vi "HFRR ADV v019 new software.vi"() -> ()   [LabVIEW 2025] (continued)
        n906 = call <vilib>:"Clear Errors.vi"("error in (no error)"=w1070) -> ("error out"=w1069:errorcluster)  [unwired: 5 in, 1 out]
        n907 = call "IMAGE ANALYSIS.vi"("Enum"=POST_ANALYSIS_ENUM."SHOW UI", "error in"=w1069) -> ("error out"=w1067:errorcluster)  [unwired: 8 in, 1 out]
        n908 = local write "Zoom Factore"(100.0 ("Zoom Factore")) -> ()
      }
    }
    n909 = case shown="True" w758 {
      selector: w758 -> [_ w1046]
      tunnel: w750 -> [w1043 w1051]
      tunnel: [w1043 w1045] -> _
      frame False {
      }
      frame True {
        n910 = Not(x=w1046) -> (.not. x?=w1044:bool)
        n911 = local read "Zoom Factore"() -> (w1049:dbl)
        n912 = local write "OUT"(w1044) -> ()
        n913 = call "IMAGE ANALYSIS.vi"("Enum"=POST_ANALYSIS_ENUM."ZOOM OUT", "error in"=w1051) -> ("error out"=w1045:errorcluster)  [unwired: 8 in, 1 out]
        n914 = Divide(x=w1049, y=1.2) -> (x/y=w1047:dbl)
        n915 = local write "Zoom Factore"(w1047) -> ()
      }
    }
    n916 = case shown="True" w759 {
      selector: w759 -> [_ w1055]
      tunnel: w750 -> [w1052 w1060]
      tunnel: [w1052 w1053] -> _
      frame False {
      }
      frame True {
        n917 = Not(x=w1055) -> (.not. x?=w1054:bool)
        n918 = local read "Zoom Factore"() -> (w1058:dbl)
        n919 = local write "In"(w1054) -> ()
        n920 = call "IMAGE ANALYSIS.vi"("Enum"=POST_ANALYSIS_ENUM."ZOOM IN", "error in"=w1060) -> ("error out"=w1053:errorcluster)  [unwired: 8 in, 1 out]
        n921 = Multiply(x=w1058, y=1.2) -> (x*y=w1056:dbl)
        n922 = local write "Zoom Factore"(w1056) -> ()
      }
    }
    n923 = case shown="True" w755 {
      selector: w755 -> [_ w1027]
      tunnel: w750 -> [w1025 w1029]
      tunnel: [w1025 w1028] -> _
      frame False {
      }
      frame True {
        n924 = Not(x=w1027) -> (.not. x?=w1026:bool)
        n925 = local write "Clear ROI Tool"(w1026) -> ()
        n926 = call "IMAGE ANALYSIS.vi"("Enum"=POST_ANALYSIS_ENUM."CLEAR ROI", "error in"=w1029) -> ("error out"=w1028:errorcluster)  [unwired: 8 in, 1 out]
      }
    }
    n927 = case shown="True" w757 {
      selector: w757 -> [_ w1039]
      tunnel: w750 -> [w1037 w1042]
      tunnel: [w1037 w1040] -> _
      frame False {
      }
      frame True {
        n928 = Not(x=w1039) -> (.not. x?=w1038:bool)
        n929 = local write "line tool"(w1038) -> ()
        n930 = call "IMAGE ANALYSIS.vi"("Enum"=POST_ANALYSIS_ENUM."DRAW LINE", "error in"=w1042) -> ("error out"=w1040:errorcluster)  [unwired: 8 in, 1 out]
      }
    }
    n931 = case shown="True" w756 {
      selector: w756 -> [_ w1033]
      tunnel: w750 -> [w1031 w1035]
      tunnel: [w1031 w1034] -> _
      frame False {
      }
      frame True {
        n932 = Not(x=w1033) -> (.not. x?=w1032:bool)
        n933 = local write "Rectangle Tool"(w1032) -> ()
        n934 = call "IMAGE ANALYSIS.vi"("Enum"=POST_ANALYSIS_ENUM."DRAW REC", "error in"=w1035) -> ("error out"=w1034:errorcluster)  [unwired: 8 in, 1 out]
      }
    }
    n935 = local read "SCAR MEASURMENT"() -> (w743:enum32{"Auto Scar", "Manual Scar"})
    n936 = local read "Fit to Screen Tool"() -> (w752:bool)
    n937 = local read "Resize Tool"() -> (w751:bool)
    n938 = case shown="\"Manual Scar\", Default" w743 {
      frame "Auto Scar" {
        n939 = property on="Cap Live Image" class="Bool (strict)"("BoolText.Text"="Report" ("Boolean Text.Text")) -> ()  [unwired: 2 in, 2 out]
      }
      frame "Manual Scar", Default {
        n940 = property on="Cap Live Image" class="Bool (strict)"("BoolText.Text"="Save Image" ("Boolean Text.Text")) -> ()  [unwired: 2 in, 2 out]
      }
    }
    n941 = local read "ROI Color Tool"() -> (w753:bool)
    n942 = local read "Pan Tool"() -> (w754:bool)
    n943 = case shown="True" w754 {
      selector: w754 -> [_ w1021]
      tunnel: w750 -> [w1019 w1023]
      tunnel: [w1019 w1022] -> _
      frame False {
      }
      frame True {
        n944 = Not(x=w1021) -> (.not. x?=w1020:bool)
        n945 = call "IMAGE ANALYSIS.vi"("Enum"=POST_ANALYSIS_ENUM."PAN", "error in"=w1023) -> ("error out"=w1022:errorcluster)  [unwired: 8 in, 1 out]
        n946 = local write "Pan Tool"(w1020) -> ()
      }
    }
    n947 = case shown="True" w751 {
      selector: w751 -> [_ w1005]
      tunnel: w750 -> [w1000 w1002]
      tunnel: [w1000 w1001] -> _
      frame False {
      }
      frame True {
        n948 = Not(x=w1005) -> (.not. x?=w1004:bool)
        n949 = local write "Resize Tool"(w1004) -> ()
        n950 = call "IMAGE ANALYSIS.vi"("Enum"=POST_ANALYSIS_ENUM."RESIZE MODE", "error in"=w1002) -> ("error out"=w1001:errorcluster)  [unwired: 8 in, 1 out]
      }
    }
    n951 = case shown="True" w752 {
      selector: w752 -> [_ w1010]
      tunnel: [w1006 w1011] -> _
      tunnel: w750 -> [w1006 w1009]
      frame False {
      }
      frame True {
        n952 = Not(x=w1010) -> (.not. x?=w1008:bool)
        n953 = local write "Zoom Factore"(100.0 ("Zoom Factore")) -> ()
        n954 = local write "Fit to Screen Tool"(w1008) -> ()
        n955 = call "IMAGE ANALYSIS.vi"("Enum"=POST_ANALYSIS_ENUM."FIT", "error in"=w1009) -> ("error out"=w1011:errorcluster)  [unwired: 8 in, 1 out]
      }
    }
    n956 = case shown="True" w753 {
      selector: w753 -> [_ w1016]
      tunnel: [w1013 w1017] -> _
      tunnel: w750 -> [w1013 w1014]
      frame False {
      }
      frame True {
        n957 = Not(x=w1016) -> (.not. x?=w1015:bool)
        n958 = local write "ROI Color Tool"(w1015) -> ()
        n959 = call "IMAGE ANALYSIS.vi"("Enum"=POST_ANALYSIS_ENUM."SET ROI COLOR", "error in"=w1014) -> ("error out"=w1017:errorcluster)  [unwired: 8 in, 1 out]
      }
    }
    n960 = local read "Quit"() -> (w767:bool)
  }
  n961 = while {
    stop <- w1101 stop-if-true
    n962 = local read "Image Path"() -> (w1104:path)
    n963 = local read "Print 3"() -> (w1107:bool)
    n964 = Equal?(x=w1104, y=path "") -> (x = y?=w1103:bool)
    n965 = Not(x=w1103) -> (.not. x?=w1102:bool)
    n966 = property on="Print 3" class="Bool (strict)"("Visible"=w1102) -> ()  [unwired: 2 in, 2 out]
    n967 = case shown="True" w1107 {
      frame False {
        n968 = local write "Rd"(TRUE ("Boolean 7")) -> ()
      }
      frame True {
        n969 = flat-sequence {
          tunnel: [w1147] -> w1115
          tunnel: [w1134] -> w1113
          tunnel: [w1144] -> w1109
          tunnel: w1115 -> [w1156]
          tunnel: [w1156] -> w1114
          tunnel: w1113 -> [w1155]
          tunnel: [w1155] -> w1112
          tunnel: [w1153] -> w1111
          tunnel: [w1152] -> w1110
          tunnel: w1109 -> [w1152]
          tunnel: w1114 -> [w1158]
          tunnel: w1112 -> [w1159]
          tunnel: w1111 -> [_]
          tunnel: w1110 -> [w1157]
          frame #0 {
            n970 = case shown="True" "Rd" {
              frame False {
              }
              frame True {
                n971 = while {
                  tunnel: "abcdefABCDEF" ("string 2") -> [w1126]
                  shift-right: [w1124] -> w1118
                  shift-left: "" -> [w1123]
                  i -> [w1133]
                  stop <- w1132 stop-if-true
                  n972 = Random Number (0-1)() -> (number: 0 to 1=w1127:dbl)
                  n973 = Multiply(x=w1127, y=62.0) -> (x*y=w1129:dbl)
                  n974 = Decrement(x="Length 2") -> (x-1=w1122:i16)
                  n975 = To Word Integer(number=w1129) -> (16bit integer=w1130:i16)
                  n976 = String Subset(string=w1126, offset (0)=w1130, length (rest)=1 ("length (rest)")) -> (substring=w1125:string)
                  n977 = Greater Or Equal?(x=w1133, y=w1122) -> (x >= y?=w1132:bool)
                  n978 = Concatenate Strings(w1125, w1123) -> (w1124:string)
                }
                "String 10" <- w1118
                n979 = local write "Rd"(FALSE ("Boolean 7")) -> ()
              }
            }
          }
          frame #1 {
            w1145 = "_resized.jpg" ("command line")
            (unwired) ".jpg -resize 320x240 " ("string")
            (unwired) "Choose an Image File" ("prompt")
            # "-resize 1798x425"
            n980 = local read "Image Path"() -> (w1139:path)
            n981 = Strip Path(path=w1139) -> (stripped path=w1134:path, name=w1135:string)
            n982 = Match Pattern(string=w1135, regular expression=".jpg") -> (before substring=→"before substring 2":string, after substring=→"after substring":string)  [unwired: 1 in, 2 out]
            n983 = Match Pattern(string=w1135, regular expression="\\") -> (before substring=w1141:string)  [unwired: 1 in, 3 out]
            n984 = Match Pattern(string=w1141, regular expression=".jpg") -> (before substring=w1140:string)  [unwired: 1 in, 3 out]
            n985 = Concatenate Strings("cmd /c convert " ("string"), w1140, ".jpg -resize 320x240  " ("command line"), w1140, w1145) -> (w1148:string)
            n986 = call <vilib>:"System Exec.vi"("run minimized? (F)"=TRUE, "wait until completion? (T)"=TRUE, "working directory"=w1134, "command line"=w1148) -> ("error out"=w1147:errorcluster)  [unwired: 4 in, 3 out]
            "error out 2" <- w1147
            n987 = Concatenate Strings(w1140, w1145) -> (w1144:string)
          }
          frame #2 {
            n988 = Wait (ms)(milliseconds to wait=u32 2000 ("millisecond timer value")) -> (millisecond timer value=w1153:u32)
          }
          frame #3 {
            n989 = case shown="No Error" w1158 {
              tunnel: w1159 -> [w1162 _]
              tunnel: w1157 -> [w1160 _]
              frame No Error {
                (unwired) ".jpg" ("string")
                n990 = Path To String(path=w1162) -> (string=w1166:string)
                n991 = Concatenate Strings(w1166, "\\" ("string"), w1160) -> (w1165:string)
                n992 = String To Path(string=w1165) -> (path=w1164:path)
                n993 = call <vilib>:"Read JPEG File.vi"("path to JPEG file"=w1164) -> ("image data"=w1168:T16)  [unwired: 8 in, 2 out]
                "image data" <- w1168
                n994 = local write "Print 3"(FALSE ("Print 2")) -> ()
                n995 = call <vilib>:"Draw Flattened Pixmap.vi"("image data"=w1168) -> ("new picture"=→"new picture":picture)  [unwired: 8 in]
              }
              frame Error {
              }
            }
          }
        }
      }
    }
    n996 = Wait (ms)(milliseconds to wait=u32 20 ("millisecond timer value")) -> ()  [unwired: 1 out]
    n997 = local read "Quit"() -> (w1101:bool)
  }
  n998 = while {
    tunnel: w35 -> [_]
    tunnel: w19 -> [_]
    stop <- w1199 stop-if-true
    # "New Adv Logics"
    n999 = local read "Main Tab"() -> (w1179:T2)
    n1000 = local read "Main Tab"() -> (w1197:T2)
    n1001 = local read "Sign In"() -> (w1196:bool)
    n1002 = case shown="\"Adv Scar\"" w1179 {
      frame "HOME", Default {
        n1003 = local read "LIVE FEED MIN TEMP"() -> (w1332:bool)
        n1004 = local write "LIVE FEED MAX TEMP"(TRUE ("LIVE FEED MAX TEMP")) -> ()
        n1005 = local read "CAMERA ROI MIN TEMP"() -> (w1330:bool)
        n1006 = case shown="True" w1332 {
          selector: w1332 -> [_ w1339]
          frame False {
          }
          frame True {
            n1007 = Not(x=w1339) -> (.not. x?=w1338:bool)
            n1008 = local write "LIVE FEED MIN TEMP"(w1338) -> ()
            n1009 = call "CAMERA LIVE FEED FGV.vi"("Enum - Menu"=CAMERA_LIVE_FEED_ENUM."CAMERA MINIMIZE") -> ()  [unwired: 9 in, 2 out]
          }
        }
        n1010 = case shown="True" w1330 {
          selector: w1330 -> [_ w1336]
          frame False {
          }
          frame True {
            n1011 = Not(x=w1336) -> (.not. x?=w1335:bool)
            n1012 = local write "CAMERA ROI MIN TEMP"(w1335) -> ()
            n1013 = call "IMAGE ANALYSIS.vi"("Enum"=POST_ANALYSIS_ENUM."MINIMIZE UI") -> ()  [unwired: 9 in, 2 out]
          }
        }
        n1014 = local write "CAMERA ROI MAX TEMP"(TRUE ("CAMERA ROI MAX TEMP")) -> ()
      }
      frame "Test Setup" {
        n1015 = local read "LIVE FEED MIN TEMP"() -> (w1342:bool)
        n1016 = local read "CAMERA ROI MIN TEMP"() -> (w1340:bool)
        n1017 = local write "LIVE FEED MAX TEMP"(TRUE ("LIVE FEED MAX TEMP")) -> ()
        n1018 = case shown="True" w1342 {
          selector: w1342 -> [_ w1349]
          frame False {
          }
          frame True {
            n1019 = Not(x=w1349) -> (.not. x?=w1348:bool)
            n1020 = local write "LIVE FEED MIN TEMP"(w1348) -> ()
            n1021 = call "CAMERA LIVE FEED FGV.vi"("Enum - Menu"=CAMERA_LIVE_FEED_ENUM."CAMERA MINIMIZE") -> ()  [unwired: 9 in, 2 out]
          }
        }
        n1022 = case shown="True" w1340 {
          selector: w1340 -> [_ w1346]
          frame False {
          }
          frame True {
            n1023 = Not(x=w1346) -> (.not. x?=w1345:bool)
            n1024 = local write "CAMERA ROI MIN TEMP"(w1345) -> ()
            n1025 = call "IMAGE ANALYSIS.vi"("Enum"=POST_ANALYSIS_ENUM."MINIMIZE UI") -> ()  [unwired: 9 in, 2 out]
          }
        }
        n1026 = local write "CAMERA ROI MAX TEMP"(TRUE ("CAMERA ROI MAX TEMP")) -> ()
      }
      frame "Acquire" {
        n1027 = local read "LIVE FEED MIN TEMP"() -> (w1352:bool)
        n1028 = local write "LIVE FEED MAX TEMP"(TRUE ("LIVE FEED MAX TEMP")) -> ()
        n1029 = local read "CAMERA ROI MIN TEMP"() -> (w1350:bool)
        n1030 = case shown="True" w1352 {
          selector: w1352 -> [_ w1359]
          frame False {
          }
          frame True {
            n1031 = Not(x=w1359) -> (.not. x?=w1358:bool)
            n1032 = local write "LIVE FEED MIN TEMP"(w1358) -> ()
            n1033 = call "CAMERA LIVE FEED FGV.vi"("Enum - Menu"=CAMERA_LIVE_FEED_ENUM."CAMERA MINIMIZE") -> ()  [unwired: 9 in, 2 out]
          }
        }
        n1034 = case shown="True" w1350 {
          selector: w1350 -> [_ w1356]
          frame False {
          }
          frame True {
            n1035 = Not(x=w1356) -> (.not. x?=w1355:bool)
            n1036 = local write "CAMERA ROI MIN TEMP"(w1355) -> ()
            n1037 = call "IMAGE ANALYSIS.vi"("Enum"=POST_ANALYSIS_ENUM."MINIMIZE UI") -> ()  [unwired: 9 in, 2 out]
          }
        }
        n1038 = local write "CAMERA ROI MAX TEMP"(TRUE ("CAMERA ROI MAX TEMP")) -> ()
      }
      frame "Adv Scar" {
        n1039 = local read "CAMERA ROI MIN TEMP"() -> (w1360:bool)
        n1040 = case shown="True" "LIVE FEED MAX TEMP" {
          selector: "LIVE FEED MAX TEMP" -> [_ w1381]
          frame False {
          }
          frame True {
            n1041 = Not(x=w1381) -> (.not. x?=w1380:bool)
            n1042 = local write "LIVE FEED MAX TEMP"(w1380) -> ()
            n1043 = call "CAMERA LIVE FEED FGV.vi"("Enum - Menu"=CAMERA_LIVE_FEED_ENUM."CAMERA RESTORE") -> ("error out"=w1371:errorcluster)  [unwired: 9 in, 1 out]
            n1044 = Type Cast(type=30, x=0) -> (*(type *) &x=w1375:i32)
            n1045 = Add(x=w1375, y=48) -> (x+y=w1376:i32)
            n1046 = call "CAMERA LIVE FEED FGV.vi"("Enum - Menu"=CAMERA_LIVE_FEED_ENUM."CAMERA MODE SET", "error in (no error)"=w1371, "CAMERA MODE"=w1376) -> ("error out"=w1368:errorcluster)  [unwired: 7 in, 1 out]
            n1047 = call "CAMERA LIVE FEED FGV.vi"("Enum - Menu"=CAMERA_LIVE_FEED_ENUM."CAMERA GRAY", "error in (no error)"=w1368) -> ("error out"=w1367:errorcluster)  [unwired: 8 in, 1 out]
            n1048 = call "LIST FILE NAMES.vi"("error in (no error)"=w1367) -> ("error out"=w1377:errorcluster, "filenames"=w1378:string[])  [unwired: 9 in]
            n1049 = property on="FILE 3" class="CmbBox"(error in=w1377, "Strings[]"=w1378) -> ()  [unwired: 1 in, 2 out]
          }
        }
        n1050 = case shown="True" w1360 {
          selector: w1360 -> [_ w1366]
          frame False {
          }
          frame True {
            n1051 = Not(x=w1366) -> (.not. x?=w1365:bool)
            n1052 = local write "CAMERA ROI MIN TEMP"(w1365) -> ()
            n1053 = call "IMAGE ANALYSIS.vi"("Enum"=POST_ANALYSIS_ENUM."MINIMIZE UI") -> ()  [unwired: 9 in, 2 out]
          }
        }
        n1054 = local write "CAMERA ROI MAX TEMP"(TRUE ("CAMERA ROI MAX TEMP")) -> ()
        "LIVE FEED MIN TEMP" <- TRUE ("LIVE FEED MIN TEMP")
      }
      frame "Adv Scar Report" {
        n1055 = local read "CAMERA ROI MAX TEMP"() -> (w1382:bool)
        n1056 = local read "LIVE FEED MIN TEMP"() -> (w1384:bool)
        n1057 = local write "LIVE FEED MAX TEMP"(TRUE ("LIVE FEED MAX TEMP")) -> ()
        n1058 = case shown="True" w1384 {
          selector: w1384 -> [_ w1393]
          frame False {
          }
          frame True {
            n1059 = Not(x=w1393) -> (.not. x?=w1392:bool)
            n1060 = local write "LIVE FEED MIN TEMP"(w1392) -> ()
            n1061 = call "CAMERA LIVE FEED FGV.vi"("Enum - Menu"=CAMERA_LIVE_FEED_ENUM."CAMERA MINIMIZE") -> ()  [unwired: 9 in, 2 out]
          }
        }
        n1062 = case shown="True" w1382 {
          selector: w1382 -> [_ w1390]
          frame False {
          }
          frame True {
            n1063 = Not(x=w1390) -> (.not. x?=w1388:bool)
            n1064 = local write "CAMERA ROI MAX TEMP"(w1388) -> ()
            n1065 = call "IMAGE ANALYSIS.vi"("Enum"=POST_ANALYSIS_ENUM."SHOW UI") -> ("error out"=w1387:errorcluster)  [unwired: 9 in, 1 out]
            n1066 = call "LIST FILE NAMES.vi"("error in (no error)"=w1387) -> ("filenames"=w1386:string[])  [unwired: 9 in, 1 out]
            n1067 = property on="Test File List :" class="CmbBox"("Strings[]"=w1386) -> ()  [unwired: 2 in, 2 out]
          }
        }
        n1068 = local write "CAMERA ROI MIN TEMP"(TRUE ("CAMERA ROI MIN TEMP")) -> ()
      }
      frame "Compare Files" {
        n1069 = local read "LIVE FEED MIN TEMP"() -> (w1396:bool)
        n1070 = local write "LIVE FEED MAX TEMP"(TRUE ("LIVE FEED MAX TEMP")) -> ()
        n1071 = local read "CAMERA ROI MIN TEMP"() -> (w1394:bool)
        n1072 = case shown="True" w1396 {
          selector: w1396 -> [_ w1403]
          frame False {
          }
          frame True {
            n1073 = Not(x=w1403) -> (.not. x?=w1402:bool)
            n1074 = local write "LIVE FEED MIN TEMP"(w1402) -> ()
            n1075 = call "CAMERA LIVE FEED FGV.vi"("Enum - Menu"=CAMERA_LIVE_FEED_ENUM."CAMERA MINIMIZE") -> ()  [unwired: 9 in, 2 out]
          }
        }
        n1076 = case shown="True" w1394 {
          selector: w1394 -> [_ w1400]
          frame False {
          }
          frame True {
            n1077 = Not(x=w1400) -> (.not. x?=w1399:bool)
            n1078 = local write "CAMERA ROI MIN TEMP"(w1399) -> ()
            n1079 = call "IMAGE ANALYSIS.vi"("Enum"=POST_ANALYSIS_ENUM."MINIMIZE UI") -> ()  [unwired: 9 in, 2 out]
          }
        }
        n1080 = local write "CAMERA ROI MAX TEMP"(TRUE ("CAMERA ROI MAX TEMP")) -> ()
      }
      frame "About" {
        n1081 = local read "LIVE FEED MIN TEMP"() -> (w1406:bool)
        n1082 = local write "LIVE FEED MAX TEMP"(TRUE ("LIVE FEED MAX TEMP")) -> ()
        n1083 = local read "CAMERA ROI MIN TEMP"() -> (w1405:bool)
        n1084 = case shown="True" w1406 {
          selector: w1406 -> [_ w1413]
          frame False {
          }
          frame True {
            n1085 = Not(x=w1413) -> (.not. x?=w1412:bool)
            n1086 = local write "LIVE FEED MIN TEMP"(w1412) -> ()
            n1087 = call "CAMERA LIVE FEED FGV.vi"("Enum - Menu"=CAMERA_LIVE_FEED_ENUM."CAMERA MINIMIZE") -> ()  [unwired: 9 in, 2 out]
          }
        }
        n1088 = case shown="True" w1405 {
          selector: w1405 -> [_ w1410]
          frame False {
          }
          frame True {
            n1089 = Not(x=w1410) -> (.not. x?=w1409:bool)
            n1090 = local write "CAMERA ROI MIN TEMP"(w1409) -> ()
            n1091 = call "IMAGE ANALYSIS.vi"("Enum"=POST_ANALYSIS_ENUM."MINIMIZE UI") -> ()  [unwired: 9 in, 2 out]
          }
        }
        n1092 = local write "CAMERA ROI MAX TEMP"(TRUE ("CAMERA ROI MIN TEMP")) -> ()
      }
      frame "Advance" {
        n1093 = local read "LIVE FEED MIN TEMP"() -> (w1416:bool)
        n1094 = local write "LIVE FEED MAX TEMP"(TRUE ("LIVE FEED MAX TEMP")) -> ()
        n1095 = local read "CAMERA ROI MIN TEMP"() -> (w1414:bool)
        n1096 = case shown="True" w1416 {
          selector: w1416 -> [_ w1423]
          frame False {
          }
          frame True {
            n1097 = Not(x=w1423) -> (.not. x?=w1422:bool)
            n1098 = local write "LIVE FEED MIN TEMP"(w1422) -> ()
            n1099 = call "CAMERA LIVE FEED FGV.vi"("Enum - Menu"=CAMERA_LIVE_FEED_ENUM."CAMERA MINIMIZE") -> ()  [unwired: 9 in, 2 out]
          }
        }
        n1100 = local write "CAMERA ROI MAX TEMP"(TRUE ("CAMERA ROI MAX TEMP")) -> ()
        n1101 = case shown="True" w1414 {
          selector: w1414 -> [_ w1420]
          frame False {
          }
          frame True {
            n1102 = Not(x=w1420) -> (.not. x?=w1419:bool)
            n1103 = local write "CAMERA ROI MIN TEMP"(w1419) -> ()
            n1104 = call "IMAGE ANALYSIS.vi"("Enum"=POST_ANALYSIS_ENUM."MINIMIZE UI") -> ()  [unwired: 9 in, 2 out]
          }
        }
      }
      frame "Mooha" {
        n1105 = local read "LIVE FEED MIN TEMP"() -> (w1426:bool)
        n1106 = local write "LIVE FEED MAX TEMP"(TRUE ("LIVE FEED MAX TEMP")) -> ()
        n1107 = local read "CAMERA ROI MIN TEMP"() -> (w1424:bool)
        n1108 = case shown="True" w1426 {
          selector: w1426 -> [_ w1433]
          frame False {
          }
          frame True {
            n1109 = Not(x=w1433) -> (.not. x?=w1432:bool)
            n1110 = local write "LIVE FEED MIN TEMP"(w1432) -> ()
            n1111 = call "CAMERA LIVE FEED FGV.vi"("Enum - Menu"=CAMERA_LIVE_FEED_ENUM."CAMERA MINIMIZE") -> ()  [unwired: 9 in, 2 out]
          }
        }
        n1112 = local write "CAMERA ROI MAX TEMP"(TRUE ("CAMERA ROI MAX TEMP")) -> ()
        n1113 = case shown="True" w1424 {
          selector: w1424 -> [_ w1430]
          frame False {
          }
          frame True {
            n1114 = Not(x=w1430) -> (.not. x?=w1429:bool)
            n1115 = local write "CAMERA ROI MIN TEMP"(w1429) -> ()
            n1116 = call "IMAGE ANALYSIS.vi"("Enum"=POST_ANALYSIS_ENUM."MINIMIZE UI") -> ()  [unwired: 9 in, 2 out]
          }
        }
      }
    }
    n1117 = local read "Auto Start Test"() -> (w1170:bool)
    n1118 = case shown="True" "sign in temp" {
      frame False {
      }
      frame True {
        w1206 = 1 ("y")
        n1119 = local read "USERNAME"() -> (w1212:string)
        n1120 = local read "USER ID"() -> (w1209:string)
        n1121 = call <vilib>:"Trim Whitespace.vi"("string"=w1212) -> ("trimmed string"=w1211:string)  [unwired: 1 in]
        n1122 = call <vilib>:"Trim Whitespace.vi"("string"=w1209) -> ("trimmed string"=w1210:string)  [unwired: 1 in]
        n1123 = String Length(string=w1211) -> (length=w1208:i32)
        n1124 = String Length(string=w1210) -> (length=w1207:i32)
        n1125 = Greater?(x=w1208, y=w1206) -> (0:w1205:bool)
        n1126 = Greater?(x=w1207, y=w1206) -> (0:w1204:bool)
        n1127 = And(x=w1205, y=w1204) -> (x .and. y?=w1203:bool)
        n1128 = case shown="True" w1203 {
          frame False {
            n1129 = property on="Sign In" class="Bool (strict)"("DisabledEnum"=T19."Disabled" ("Disabled")) -> ()  [unwired: 2 in, 2 out]
          }
          frame True {
            n1130 = property on="Sign In" class="Bool (strict)"("DisabledEnum"=T19."Enabled" ("Disabled")) -> ()  [unwired: 2 in, 2 out]
          }
        }
      }
    }
    n1131 = local read "Air Temperature"() -> (w1187:bool)
    n1132 = local read "Coefficient Of Friction"() -> (w1188:bool)
    n1133 = case shown="False" w1170 {
      frame False {
        n1134 = local read "Auto stop temp"() -> (w1200:bool)
        n1135 = case shown="True" w1200 {
          frame False {
          }
          frame True {
            n1136 = local write "Auto Start Temp"(FALSE ("Auto Start Temp")) -> ()
          }
        }
      }
      frame True {
        "Auto stop temp" <- TRUE ("Auto stop temp")
      }
    }
    n1137 = local read "Humidity"() -> (w1186:bool)
    n1138 = case shown="\"HOME\"" w1197 {
      frame "HOME" {
        n1139 = local write "main tab sub"(enum32{"Page 1", "Page 2"}."Page 1" ("main tab sub")) -> ()
      }
      frame Default {
        n1140 = local write "main tab sub"(enum32{"Page 1", "Page 2"}."Page 2" ("main tab sub")) -> ()
      }
    }
    n1141 = case shown="True" w1196 {
      selector: w1196 -> [_ w1547]
      frame False {
      }
      frame True {
        n1142 = Not(x=w1547) -> (.not. x?=w1546:bool)
        n1143 = local write "Sign In"(w1546) -> ()
        n1144 = local write "Main Dashboard Buttons"(T24."Test Setup" ("Main Dashboard Buttons")) -> ()
      }
    }
    n1145 = case shown="\"Numeric Display\", Default" "Num/Graph" {
      frame "Numeric Display", Default {
        n1146 = property on="Single/Multiple" class="RadioBtnsControl (strict)"("Visible"=FALSE) -> ()  [unwired: 2 in, 2 out]
        n1147 = property on="Single - Graph" class="Ring (strict)"("Visible"=FALSE) -> ()  [unwired: 2 in, 2 out]
        n1148 = local write "Main Tab Display"(T4."Dashboard 1" ("Main Tab Display")) -> ()
      }
      frame "Graph Display" {
        n1149 = property on="Single/Multiple" class="RadioBtnsControl (strict)"("Visible"=TRUE) -> ()  [unwired: 2 in, 2 out]
        n1150 = case shown="\"Multiple\"" "Single/Multiple" {
          frame "Single ", Default {
            n1151 = property on="Single - Graph" class="Ring (strict)"("Visible"=TRUE) -> ()  [unwired: 2 in, 2 out]
            n1152 = local write "Main Tab Display"(T4."Dashboard 3" ("Main Tab Display")) -> ()
          }
          frame "Multiple" {
            n1153 = property on="Single - Graph" class="Ring (strict)"("Visible"=FALSE) -> ()  [unwired: 2 in, 2 out]
            n1154 = local write "Main Tab Display"(T4."Dashboard 2" ("Main Tab Display")) -> ()
          }
        }
      }
    }
    n1155 = local read "Stroke"() -> (w1185:bool)
    n1156 = local read "USERNAME"() -> (w1191:string)
    n1157 = local read "USER ID"() -> (w1190:string)
    n1158 = case shown="True" w1188 {
      selector: w1188 -> [_ w1473]
      frame False {
      }
      frame True {
        n1159 = Not(x=w1473) -> (.not. x?=w1472:bool)
        n1160 = local write "Coefficient Of Friction"(w1472) -> ()
        n1161 = local write "Tab Control 2"(T6."Coefficient Of Friction" ("Tab Control 2")) -> ()
      }
    }
    n1162 = case shown="True" w1187 {
      selector: w1187 -> [_ w1470]
      frame False {
      }
      frame True {
        n1163 = Not(x=w1470) -> (.not. x?=w1468:bool)
        n1164 = local write "Air Temperature"(w1468) -> ()
        n1165 = local write "Tab Control 2"(T6."Air Temperature" ("Tab Control 2")) -> ()
      }
    }
    n1166 = local write "Operator ID"(w1190) -> ()
    n1167 = case shown="True" w1185 {
      selector: w1185 -> [_ w1464]
      frame False {
      }
      frame True {
        n1168 = Not(x=w1464) -> (.not. x?=w1462:bool)
        n1169 = local write "Stroke"(w1462) -> ()
        n1170 = local write "Tab Control 2"(T6."Stroke" ("Tab Control 2")) -> ()
      }
    }
    n1171 = local write "tested by"(w1191) -> ()
    n1172 = case shown="True" w1186 {
      selector: w1186 -> [_ w1467]
      frame False {
      }
      frame True {
        n1173 = Not(x=w1467) -> (.not. x?=w1465:bool)
        n1174 = local write "Humidity"(w1465) -> ()
        n1175 = local write "Tab Control 2"(T6."Humidity" ("Tab Control 2")) -> ()
      }
    }
    n1176 = case shown="\"Calibration\"" "Main Dashboard Buttons" {
      tunnel: [T2."HOME" ("Main Tab") T2."Test Setup" ("Main Tab") T2."Acquire" ("Main Tab") T2."Adv Scar" ("Main Tab") T2."Adv Scar Report" ("Main Tab") T2."Compare Files" ("Main Tab") T2."Calibration" ("Main Tab") T2."About" ("Main Tab") T2."Advance" ("Main Tab")] -> w1169
      frame "Home", Default {
      }
      frame "Test Setup" {
      }
      frame "Dashboard" {
      }
      frame "Imaging" {
      }
      frame "Report" {
      }
      frame "Analysis" {
      }
      frame "Calibration" {
      }
      frame "About" {
      }
      frame "Advance" {
      }
    }
    n1177 = Wait (ms)(milliseconds to wait=u32 100) -> ()  [unwired: 1 out]
    n1178 = local read "Main Tab Display"() -> (w1189:T4)
    n1179 = local write "Main Tab"(w1169) -> ()
    n1180 = case shown="\"Dashboard 3\"" w1189 {
      frame "Dashboard 1", Default {
        n1181 = property on="Reset Graph" class="Bool (strict)"("Visible"=FALSE) -> ()  [unwired: 2 in, 2 out]
      }
      frame "Dashboard 2" {
        n1182 = property on="Reset Graph" class="Bool (strict)"("Visible"=TRUE) -> ()  [unwired: 2 in, 2 out]
      }
      frame "Dashboard 3" {
        n1183 = property on="Reset Graph" class="Bool (strict)"("Visible"=TRUE) -> ()  [unwired: 2 in, 2 out]
      }
    }
    n1184 = local read "SCAR MEASURMENT"() -> (w1177:enum32{"Auto Scar", "Manual Scar"})
    n1185 = local read "Humidity"() -> (w1192:bool)
    n1186 = local read "Cap Live Image"() -> (w1174:bool)
    n1187 = local read "Sample Temperature"() -> (w1184:bool)
    n1188 = local read "Air Temp vs Humidity"() -> (w1182:bool)
    n1189 = local read "Frequency"() -> (w1183:bool)
    n1190 = case shown="True" w1192 {
      frame False {
        n1191 = local write "Humidity On Command"(TRUE ("Humidity On Command")) -> ()
        n1192 = case shown="True" "Humidity Off Command" {
          selector: "Humidity Off Command" -> [_ w1480]
          frame False {
          }
          frame True {
            n1193 = stacked-sequence {
              frame #0 {
                n1194 = local read "WriteHumidity 2"() -> (w1482:string[])
                n1195 = Insert Into Array(array=w1482, new element="R;1" ("new element/subarray")) -> (w1481:string[])  [unwired: 1 in]
                n1196 = local write "WriteHumidity 2"(w1481) -> ()
              }
              frame #1 {
                n1197 = Wait (ms)(milliseconds to wait=u32 2000) -> ()  [unwired: 1 out]
              }
              frame #2 {
                n1198 = local read "WriteHumidity 2"() -> (w1485:string[])
                n1199 = local read "EVENT LOG"() -> (w1489:string)
                n1200 = call "Event Log.vi"("Content"="Humidity Control Off" ("string"), "EVENT LOG"=w1489) -> ("EVENT LOG"=w1490:string)  [unwired: 8 in, 1 out]
                n1201 = local write "EVENT LOG"(w1490) -> ()
                n1202 = Insert Into Array(array=w1485, new element="R;1" ("new element/subarray")) -> (w1486:string[])  [unwired: 1 in]
                n1203 = local write "WriteHumidity 2"(w1486) -> ()
              }
            }
            n1204 = Not(x=w1480) -> (.not. x?=w1479:bool)
            n1205 = local write "Humidity Off Command"(w1479) -> ()
          }
        }
      }
      frame True {
        n1206 = local write "Humidity Off Command"(TRUE ("Humidity Off Command")) -> ()
        n1207 = case shown="True" "Humidity On Command" {
          selector: "Humidity On Command" -> [_ w1494]
          frame False {
          }
          frame True {
            n1208 = stacked-sequence {
              frame #0 {
                n1209 = local read "Set Rh"() -> (w1500:dbl)
                n1210 = local read "WriteHumidity 2"() -> (w1495:string[])
                n1211 = Number To Fractional String(number=w1500, precision (6)=i16 2) -> (F-format string=w1501:string)  [unwired: 2 in]
                n1212 = Concatenate Strings("M;" ("new element/subarray"), w1501) -> (w1499:string)
                n1213 = Insert Into Array(array=w1495, new element=w1499) -> (w1496:string[])  [unwired: 1 in]
                n1214 = local write "WriteHumidity 2"(w1496) -> ()
              }
              frame #1 {
                n1215 = Wait (ms)(milliseconds to wait=u32 2000) -> ()  [unwired: 1 out]
              }
              frame #2 {
                n1216 = local read "Set Rh"() -> (w1508:dbl)
                n1217 = local read "WriteHumidity 2"() -> (w1503:string[])
                n1218 = Number To Fractional String(number=w1508, precision (6)=i16 2) -> (F-format string=w1509:string)  [unwired: 2 in]
                n1219 = Concatenate Strings("M;" ("new element/subarray"), w1509) -> (w1507:string)
                n1220 = Insert Into Array(array=w1503, new element=w1507) -> (w1504:string[])  [unwired: 1 in]
                n1221 = local write "WriteHumidity 2"(w1504) -> ()
              }
              frame #3 {
                n1222 = Wait (ms)(milliseconds to wait=u32 1500) -> ()  [unwired: 1 out]
              }
              frame #4 {
                (unwired) "% RH" ("string")
                (unwired) i16 2 ("precision (6)")
                (unwired) "M;" ("new element/subarray")
                n1223 = local read "Set Rh"() -> (w1518:dbl)
                n1224 = local read "WriteHumidity 2"() -> (w1511:string[])
                n1225 = Number To Fractional String(number=w1518, precision (6)=i16 2) -> (F-format string=w1515:string)  [unwired: 2 in]
                n1226 = Concatenate Strings("M;" ("new element/subarray"), w1515) -> (w1519:string)
                n1227 = Concatenate Strings("Humidity Set to : " ("string"), w1515, "% RH" ("string")) -> (w1513:string)
                n1228 = Insert Into Array(array=w1511, new element=w1519) -> (w1512:string[])  [unwired: 1 in]
                n1229 = disable-structure shown="Enabled" {
                  frame Enabled {
                    n1230 = local read "EVENT LOG"() -> (w1522:string)
                    n1231 = call "Event Log.vi"("Content"="Humidity Control On", "EVENT LOG"=w1522) -> ("EVENT LOG"=w1523:string)  [unwired: 8 in, 1 out]
                    n1232 = local write "EVENT LOG"(w1523) -> ()
                  }
                  frame Disabled {
                  }
                }
                n1233 = disable-structure shown="Enabled" {
                  disable-tunnel: w1513 -> [_ _]
                  frame Enabled {
                    n1234 = local read "EVENT LOG"() -> (w1525:string)
                    n1235 = call "Event Log.vi"("Content"="Humidity Control On", "EVENT LOG"=w1525) -> ("EVENT LOG"=w1526:string)  [unwired: 8 in, 1 out]
                    n1236 = local write "EVENT LOG"(w1526) -> ()
                  }
                  frame Disabled {
                  }
                }
                n1237 = local write "WriteHumidity 2"(w1512) -> ()
              }
            }
            n1238 = Not(x=w1494) -> (.not. x?=w1493:bool)
            n1239 = local write "Humidity On Command"(w1493) -> ()
          }
        }
      }
    }
    n1240 = Equal?(x=w1177, y=enum32{"Auto Scar", "Manual Scar"}."Auto Scar" ("SCAR MEASURMENT")) -> (x = y?=w1173:bool)
    n1241 = local read "TEST STANDARD"() -> (w1180:T3)
    n1242 = And(x=w1174, y=w1173) -> (x .and. y?=w1175:bool)
    n1243 = case shown="True" w1175 {
      selector: w1175 -> [_ w1279]
      tunnel: errorcluster {"status"=FALSE, "code"=0, "source"=""} ("error in (no error) 3") -> [_ w1280]
      frame False {
      }
      frame True {
        n1244 = stacked-sequence {
          tunnel: w1280 -> [_ _ _ _ _ _ _ w1328]
          tunnel: w1279 -> [_ _ _ _ _ w1309 _ _]
          frame #0 {
            n1245 = call "CAMERA LIVE FEED FGV.vi"("Enum - Menu"=CAMERA_LIVE_FEED_ENUM."CAMERA MINIMIZE") -> ()  [unwired: 9 in, 2 out]
          }
          frame #1 {
            n1246 = property on="Auto Scar Check  2" class="Clust (strict)"("Visible"=TRUE) -> ()  [unwired: 2 in, 2 out]
          }
          frame #2 {
            n1247 = String To Path(string="C:\\LAB-IQ\\Image Calibrate v01.dcf") -> (path=w1285:path)
            n1248 = Open/Create/Replace File ("Open File")(file path (use dialog)=w1285) -> (refnum out=w1286:refnum<file>)  [unwired: 5 in, 2 out]
            n1249 = for {
              N: 4 -> [_]
              tunnel: w1286 -> [w1292]
              i -> [w1288]
              n1250 = Read from Text File ("Read File")(file (use dialog)=w1292) -> (text=w1293:string)  [unwired: 3 in, 3 out]
              n1251 = String Subset(string=w1293, offset (0)=6, length (rest)=10 ("length (rest)")) -> (substring=w1289:string)
              n1252 = Fract/Exp String To Number(string=w1289) -> (number=w1287:dbl)  [unwired: 3 in, 1 out]
              n1253 = case shown="0" w1288 {
                tunnel: w1287 -> [w1294 w1295 _ w1296 _]
                frame 0 {
                  "5x Gain" <- w1294
                }
                frame 1 {
                  "10x Gain" <- w1295
                }
                frame 2 {
                }
                frame 3 {
                  "100x gain" <- w1296
                }
                frame 4, Default {
                }
              }
            }
          }
          frame #3 {
            n1254 = local read "FILE 3"() -> (w1302:string)
            n1255 = call <vilib>:"Trim Whitespace.vi"("string"="C:\\LAB-IQ\\images\\") -> ("trimmed string"=w1304:string)  [unwired: 1 in]
            n1256 = String To Path(string=w1304) -> (path=w1303:path)
            n1257 = Concatenate Strings(w1302, ".png" ("string")) -> (w1301:string)
            n1258 = Build Path(base path=w1303, name or relative path=w1301) -> (appended path=w1299:path)
            "Image path" <- w1299
            n1259 = Path To String(path=w1299) -> (string=w1298:string)
            n1260 = call "CAMERA LIVE FEED FGV.vi"("Enum - Menu"=CAMERA_LIVE_FEED_ENUM."CAMERA SAVE", "Image Path"=w1298) -> ()  [unwired: 8 in, 2 out]
          }
          frame #4 {
            n1261 = One Button Dialog(message="Image saved successfully") -> ()  [unwired: 1 in, 1 out]
          }
          frame #5 {
            n1262 = local read "TEST STANDARD"() -> (w1308:T3)
            n1263 = local read "Magnification len live scar"() -> (w1320:string)
            n1264 = Not(x=w1309) -> (.not. x?=w1310:bool)
            n1265 = local write "Cap Live Image"(w1310) -> ()
            n1266 = case shown="\"ISO 12156\"" w1308 {
              tunnel: ["ASTM D6079" "ISO 12156"] -> w1307
              frame "ASTM D6079", Default {
              }
              frame "ISO 12156" {
              }
            }
            n1267 = case shown="\"5x\", Default" w1320 {
              tunnel: [w1323 w1324] -> w1319
              frame "5x", Default {
                n1268 = local read "5x Gain"() -> (w1323:dbl)
              }
              frame "10x" {
                # "5x"
                n1269 = local read "10x Gain"() -> (w1324:dbl)
              }
            }
            n1270 = local read "Image path"() -> (w1318:path)
            n1271 = local read "FILE 3"() -> (w1311:string)
            n1272 = call "EDGE DETCTION.vi"("GAIN VALUE"=w1319, "Image Path"=w1318) -> ("error out"=w1317:errorcluster, "return value"=w1316:cluster{string, string, dbl, dbl, dbl})  [unwired: 8 in]
            n1273 = Bundle By Name(cluster=T25 {"File Name"="", "Test Method"="", "Operator"="", "Fuel Description"="", "Date and time"=""} ("Main Ref"), "File Name"=w1311, "Test Method"=w1307) -> (w1312:T25)
            n1274 = call "duf file read.vi"("error in (no error)"=w1317, "Main Ref"=w1312) -> ("error out"=w1315:errorcluster, "Main Ref 2"=w1313:T25)  [unwired: 8 in]
            n1275 = call "EDGE DETECTION REPORT.vi"("error in (no error)"=w1315, "return value 2"=w1316, "Main Ref"=w1313) -> ()  [unwired: 8 in, 1 out]
          }
          frame #6 {
            n1276 = property on="Auto Scar Check  2" class="Clust (strict)"("Visible"=FALSE) -> ()  [unwired: 2 in, 2 out]
          }
          frame #7 {
            n1277 = call "CAMERA LIVE FEED FGV.vi"("Enum - Menu"=CAMERA_LIVE_FEED_ENUM."CAMERA MINIMIZE", "error in (no error)"=w1328) -> ()  [unwired: 8 in, 2 out]
            n1278 = local write "Main Dashboard Buttons"(T1."Home" ("Main Dashboard Buttons")) -> ()
            n1279 = local write "Main Tab"(T2."HOME" ("Main Tab")) -> ()
          }
        }
      }
    }
    n1280 = local read "Heater Button"() -> (w1181:bool)
    n1281 = case shown="True" w1183 {
      selector: w1183 -> [_ w1458]
      frame False {
      }
      frame True {
        n1282 = Not(x=w1458) -> (.not. x?=w1456:bool)
        n1283 = local write "Frequency"(w1456) -> ()
        n1284 = local write "Tab Control 2"(T6."Frequency" ("Tab Control 2")) -> ()
      }
    }
    n1285 = case shown="True" w1182 {
      selector: w1182 -> [_ w1455]
      frame False {
      }
      frame True {
        n1286 = Not(x=w1455) -> (.not. x?=w1453:bool)
        n1287 = local write "Air Temp vs Humidity"(w1453) -> ()
        n1288 = local write "Tab Control 2"(T6."Air Temp vs Rh" ("Tab Control 2")) -> ()
      }
    }
    n1289 = case shown="True" w1184 {
      selector: w1184 -> [_ w1461]
      frame False {
      }
      frame True {
        n1290 = Not(x=w1461) -> (.not. x?=w1459:bool)
        n1291 = local write "Sample Temperature"(w1459) -> ()
        n1292 = local write "Tab Control 2"(T6."Sample Temperature" ("Tab Control 2")) -> ()
      }
    }
    n1293 = case shown="\"Custom\"" w1180 {
      frame "ASTM D6079", Default {
        w1434 = "ASTM D6079 TEST CONDITIONS" ("Standard 2")
        n1294 = local write "Standard 2"(w1434) -> ()
        n1295 = local write "Standard"(w1434) -> ()
      }
      frame "ISO 12156" {
        w1435 = "ISO 12156 TEST CONDITIONS" ("Standard 2")
        n1296 = local write "Standard 2"(w1435) -> ()
        n1297 = local write "Standard"(w1435) -> ()
      }
      frame "CEC F-096-A-06" {
        w1436 = "CEC F-096-A-06 TEST CONDITIONS" ("Standard 2")
        n1298 = local write "Standard 2"(w1436) -> ()
        n1299 = local write "Standard"(w1436) -> ()
      }
      frame "Custom" {
        w1437 = "CUSTOM TEST CONDITIONS" ("Standard 2")
        n1300 = local write "Standard 2"(w1437) -> ()
        n1301 = local write "Standard"(w1437) -> ()
      }
    }
    n1302 = case shown="True" w1181 {
      frame False {
        n1303 = local write "Temperature On Command"(TRUE ("Temperature On Command")) -> ()
        n1304 = case shown="True" "Temperature Off Command" {
          selector: "Temperature Off Command" -> [_ w1441]
          frame False {
          }
          frame True {
            n1305 = Not(x=w1441) -> (.not. x?=w1440:bool)
            n1306 = local read "EVENT LOG"() -> (w1444:string)
            n1307 = local write "Temperature Off Command"(w1440) -> ()
            n1308 = call "Event Log.vi"("Content"="Heater Off", "EVENT LOG"=w1444) -> ("EVENT LOG"=w1443:string)  [unwired: 8 in, 1 out]
            n1309 = local write "EVENT LOG"(w1443) -> ()
          }
        }
      }
      frame True {
        n1310 = local write "Temperature Off Command"(TRUE ("Temperature Off Command")) -> ()
        n1311 = case shown="True" "Temperature On Command" {
          selector: "Temperature On Command" -> [_ w1448]
          frame False {
          }
          frame True {
            n1312 = Not(x=w1448) -> (.not. x?=w1447:bool)
            n1313 = local write "Temperature On Command"(w1447) -> ()
            n1314 = disable-structure shown="Enabled" {
              disable-tunnel: "Heater On" -> [w1450 _]
              frame Enabled {
                n1315 = local read "EVENT LOG"() -> (w1451:string)
                n1316 = call "Event Log.vi"("Content"=w1450, "EVENT LOG"=w1451) -> ("EVENT LOG"=w1452:string)  [unwired: 8 in, 1 out]
                n1317 = local write "EVENT LOG"(w1452) -> ()
              }
              frame Disabled {
              }
            }
          }
        }
      }
    }
    n1318 = local read "Main Tab"() -> (w1172:T2)
    n1319 = case shown="\"About\"" w1172 {
      frame "HOME", Default {
        w1215 = T19."Enabled" ("Disabled")
        n1320 = local read "Service Password enable"() -> (w1217:bool)
        n1321 = property on="Imaging" class="Bool (strict)"("DisabledEnum"=w1215) -> ()  [unwired: 2 in, 2 out]
        n1322 = property on="Dashboard" class="Bool (strict)"("DisabledEnum"=w1215) -> ()  [unwired: 2 in, 2 out]
        n1323 = property on="Test Setup" class="Bool (strict)"("DisabledEnum"=w1215) -> ()  [unwired: 2 in, 2 out]
        n1324 = property on="Analysis" class="Bool (strict)"("DisabledEnum"=w1215) -> ()  [unwired: 2 in, 2 out]
        n1325 = property on="Home" class="Bool (strict)"("DisabledEnum"=w1215) -> ()  [unwired: 2 in, 2 out]
        n1326 = property on="Report" class="Bool (strict)"("DisabledEnum"=w1215) -> ()  [unwired: 2 in, 2 out]
        n1327 = property on="Main Dashboard Buttons" class="RadioBtnsControl (strict)"("DisabledEnum"=w1215) -> ()  [unwired: 2 in, 2 out]
        n1328 = property on="Calibration" class="Bool (strict)"("DisabledEnum"=w1215) -> ()  [unwired: 2 in, 2 out]
        n1329 = case shown="True" w1217 {
          tunnel: [T19."Disabled" ("Disabled") T19."Enabled" ("Disabled")] -> w1216
          frame False {
          }
          frame True {
          }
        }
        n1330 = property on="About" class="Bool (strict)"("DisabledEnum"=w1216) -> ()  [unwired: 2 in, 2 out]
      }
      frame "Test Setup" {
        w1222 = T19."Enabled" ("Disabled")
        n1331 = local read "Service Password enable"() -> (w1221:bool)
        n1332 = property on="Dashboard" class="Bool (strict)"("DisabledEnum"=T19."Disabled" ("Disabled")) -> ()  [unwired: 2 in, 2 out]
        n1333 = property on="Imaging" class="Bool (strict)"("DisabledEnum"=w1222) -> ()  [unwired: 2 in, 2 out]
        n1334 = property on="Analysis" class="Bool (strict)"("DisabledEnum"=w1222) -> ()  [unwired: 2 in, 2 out]
        n1335 = property on="Home" class="Bool (strict)"("DisabledEnum"=w1222) -> ()  [unwired: 2 in, 2 out]
        n1336 = property on="Report" class="Bool (strict)"("DisabledEnum"=w1222) -> ()  [unwired: 2 in, 2 out]
        n1337 = property on="Test Setup" class="Bool (strict)"("DisabledEnum"=w1222) -> ()  [unwired: 2 in, 2 out]
        n1338 = case shown="True" w1221 {
          tunnel: [T19."Disabled" ("Disabled") T19."Enabled" ("Disabled")] -> w1220
          frame False {
          }
          frame True {
          }
        }
        n1339 = property on="About" class="Bool (strict)"("DisabledEnum"=w1220) -> ()  [unwired: 2 in, 2 out]
      }
      frame "Adv Scar" {
        w1229 = T19."Enabled" ("Disabled")
        n1340 = property on="Dashboard" class="Bool (strict)"("DisabledEnum"=T19."Disabled" ("Disabled")) -> ()  [unwired: 2 in, 2 out]
        n1341 = property on="Imaging" class="Bool (strict)"("DisabledEnum"=w1229) -> ()  [unwired: 2 in, 2 out]
        n1342 = property on="Analysis" class="Bool (strict)"("DisabledEnum"=w1229) -> ()  [unwired: 2 in, 2 out]
        n1343 = property on="Home" class="Bool (strict)"("DisabledEnum"=w1229) -> ()  [unwired: 2 in, 2 out]
        n1344 = property on="Report" class="Bool (strict)"("DisabledEnum"=w1229) -> ()  [unwired: 2 in, 2 out]
        n1345 = property on="Test Setup" class="Bool (strict)"("DisabledEnum"=w1229) -> ()  [unwired: 2 in, 2 out]
        n1346 = local read "Service Password enable"() -> (w1227:bool)
        n1347 = case shown="True" w1227 {
          tunnel: [T19."Disabled" ("Disabled") T19."Enabled" ("Disabled")] -> w1226
          frame False {
          }
          frame True {
          }
        }
        n1348 = property on="About" class="Bool (strict)"("DisabledEnum"=w1226) -> ()  [unwired: 2 in, 2 out]
      }
      frame "Calibration" {
        w1232 = T19."Enabled" ("Disabled")
        n1349 = property on="Dashboard" class="Bool (strict)"("DisabledEnum"=T19."Disabled" ("Disabled")) -> ()  [unwired: 2 in, 2 out]
        n1350 = property on="Imaging" class="Bool (strict)"("DisabledEnum"=w1232) -> ()  [unwired: 2 in, 2 out]
        n1351 = property on="Analysis" class="Bool (strict)"("DisabledEnum"=w1232) -> ()  [unwired: 2 in, 2 out]
        n1352 = property on="Home" class="Bool (strict)"("DisabledEnum"=w1232) -> ()  [unwired: 2 in, 2 out]
        n1353 = property on="Report" class="Bool (strict)"("DisabledEnum"=w1232) -> ()  [unwired: 2 in, 2 out]
        n1354 = property on="Test Setup" class="Bool (strict)"("DisabledEnum"=w1232) -> ()  [unwired: 2 in, 2 out]
        n1355 = local read "Service Password enable"() -> (w1234:bool)
        n1356 = property on="Calibration" class="Bool (strict)"("DisabledEnum"=w1232) -> ()  [unwired: 2 in, 2 out]
        n1357 = case shown="True" w1234 {
          tunnel: [T19."Disabled" ("Disabled") T19."Enabled" ("Disabled")] -> w1233
          frame False {
          }
          frame True {
          }
        }
        n1358 = property on="About" class="Bool (strict)"("DisabledEnum"=w1233) -> ()  [unwired: 2 in, 2 out]
      }
      frame "Adv Scar Report" {
        w1240 = T19."Enabled" ("Disabled")
        n1359 = property on="Dashboard" class="Bool (strict)"("DisabledEnum"=T19."Disabled" ("Disabled")) -> ()  [unwired: 2 in, 2 out]
        n1360 = property on="Imaging" class="Bool (strict)"("DisabledEnum"=w1240) -> ()  [unwired: 2 in, 2 out]
        n1361 = property on="Analysis" class="Bool (strict)"("DisabledEnum"=w1240) -> ()  [unwired: 2 in, 2 out]
        n1362 = property on="Home" class="Bool (strict)"("DisabledEnum"=w1240) -> ()  [unwired: 2 in, 2 out]
        n1363 = property on="Report" class="Bool (strict)"("DisabledEnum"=w1240) -> ()  [unwired: 2 in, 2 out]
        n1364 = property on="Test Setup" class="Bool (strict)"("DisabledEnum"=w1240) -> ()  [unwired: 2 in, 2 out]
        n1365 = local read "Service Password enable"() -> (w1239:bool)
        n1366 = case shown="True" w1239 {
          tunnel: [T19."Disabled" ("Disabled") T19."Enabled" ("Disabled")] -> w1238
          frame False {
          }
          frame True {
          }
        }
        n1367 = property on="About" class="Bool (strict)"("DisabledEnum"=w1238) -> ()  [unwired: 2 in, 2 out]
      }
      frame "Compare Files" {
        w1246 = T19."Enabled" ("Disabled")
        n1368 = local read "Service Password enable"() -> (w1245:bool)
        n1369 = property on="Dashboard" class="Bool (strict)"("DisabledEnum"=T19."Disabled" ("Disabled")) -> ()  [unwired: 2 in, 2 out]
        n1370 = property on="Imaging" class="Bool (strict)"("DisabledEnum"=w1246) -> ()  [unwired: 2 in, 2 out]
        n1371 = property on="Analysis" class="Bool (strict)"("DisabledEnum"=w1246) -> ()  [unwired: 2 in, 2 out]
        n1372 = property on="Home" class="Bool (strict)"("DisabledEnum"=w1246) -> ()  [unwired: 2 in, 2 out]
        n1373 = property on="Report" class="Bool (strict)"("DisabledEnum"=w1246) -> ()  [unwired: 2 in, 2 out]
        n1374 = property on="Test Setup" class="Bool (strict)"("DisabledEnum"=w1246) -> ()  [unwired: 2 in, 2 out]
        n1375 = case shown="True" w1245 {
          tunnel: [T19."Disabled" ("Disabled") T19."Enabled" ("Disabled")] -> w1244
          frame False {
          }
          frame True {
          }
        }
        n1376 = property on="About" class="Bool (strict)"("DisabledEnum"=w1244) -> ()  [unwired: 2 in, 2 out]
      }
      frame "Acquire" {
        n1377 = local read "Service Password enable"() -> (w1251:bool)
        n1378 = property on="Test Setup" class="Bool (strict)"("DisabledEnum"=T19."Disabled" ("Disabled")) -> ()  [unwired: 2 in, 2 out]
        n1379 = local read "Auto Start Test"() -> (w1253:bool)
        n1380 = local read "RUN"() -> (w1255:bool)
        n1381 = case shown="True" w1251 {
          tunnel: [T19."Disabled" ("Disabled") T19."Enabled" ("Disabled")] -> w1252
          frame False {
          }
          frame True {
          }
        }
        n1382 = Or(x=w1255, y=w1253) -> (x .or. y?=w1254:bool)
        n1383 = case shown="True" w1254 {
          tunnel: [T19."Enabled" ("Disabled") T19."Disabled" ("Disabled")] -> w1250
          frame False {
          }
          frame True {
          }
        }
        n1384 = property on="About" class="Bool (strict)"("DisabledEnum"=w1252) -> ()  [unwired: 2 in, 2 out]
        n1385 = property on="Imaging" class="Bool (strict)"("DisabledEnum"=w1250) -> ()  [unwired: 2 in, 2 out]
        n1386 = property on="Dashboard" class="Bool (strict)"("DisabledEnum"=w1250) -> ()  [unwired: 2 in, 2 out]
        n1387 = property on="Analysis" class="Bool (strict)"("DisabledEnum"=w1250) -> ()  [unwired: 2 in, 2 out]
        n1388 = property on="Home" class="Bool (strict)"("DisabledEnum"=w1250) -> ()  [unwired: 2 in, 2 out]
        n1389 = property on="Report" class="Bool (strict)"("DisabledEnum"=w1250) -> ()  [unwired: 2 in, 2 out]
        n1390 = property on="Calibration" class="Bool (strict)"("DisabledEnum"=w1250) -> ()  [unwired: 2 in, 2 out]
      }
      frame "About" {
        n1391 = local read "FILE"() -> (w1269:string)
        n1392 = local read "TEST FILE NAM,E SAVED"() -> (w1262:bool)
        n1393 = call <vilib>:"Trim Whitespace.vi"("string"=w1269) -> ("trimmed string"=w1268:string)  [unwired: 1 in]
        n1394 = local read "Auto Start Test"() -> (w1272:bool)
        n1395 = String Length(string=w1268) -> (length=w1267:i32)
        n1396 = Greater?(x=w1267, y=1) -> (0:w1264:bool)
        n1397 = And(x=w1264, y=w1262) -> (x .and. y?=w1263:bool)
        n1398 = local read "RUN"() -> (w1274:bool)
        n1399 = case shown="True" w1263 {
          tunnel: [T19."Disabled" ("Disabled") T19."Enabled" ("Disabled")] -> w1265
          frame False {
          }
          frame True {
          }
        }
        n1400 = Or(x=w1274, y=w1272) -> (x .or. y?=w1273:bool)
        n1401 = property on="About" class="Bool (strict)"("DisabledEnum"=T19."Enabled" ("Disabled")) -> ()  [unwired: 2 in, 2 out]
        n1402 = case shown="False" w1273 {
          tunnel: [T19."Enabled" ("Disabled") T19."Disabled" ("Disabled")] -> w1271
          frame False {
          }
          frame True {
          }
        }
        n1403 = property on="Dashboard" class="Bool (strict)"("DisabledEnum"=w1265) -> ()  [unwired: 2 in, 2 out]
        n1404 = property on="Test Setup" class="Bool (strict)"("DisabledEnum"=T19."Disabled" ("Disabled")) -> ()  [unwired: 2 in, 2 out]
        n1405 = property on="Imaging" class="Bool (strict)"("DisabledEnum"=w1271) -> ()  [unwired: 2 in, 2 out]
        n1406 = property on="Analysis" class="Bool (strict)"("DisabledEnum"=w1271) -> ()  [unwired: 2 in, 2 out]
        n1407 = property on="Home" class="Bool (strict)"("DisabledEnum"=w1271) -> ()  [unwired: 2 in, 2 out]
        n1408 = property on="Report" class="Bool (strict)"("DisabledEnum"=w1271) -> ()  [unwired: 2 in, 2 out]
      }
    }
    n1409 = local read "Quit"() -> (w1199:bool)
    "Single" <- "Single - Graph"
  }
  n1410 = disable-structure shown="Disabled" {
    disable-tunnel: [w1551 _] -> w41
    disable-tunnel: _ -> [w1550 _]
    frame Disabled {
      n1411 = while {
        tunnel: w1550 -> [_]
        tunnel: [w1552] -> w1551
        tunnel: [w1553] -> _
        i -> [w1553]
        stop <- w1552 stop-if-true
        w1569 = u16 10 items=["1.0"=10, "1.5"=15, "2.0"=20] ("stop bits (10: 1 bit)")
        n1412 = Wait (ms)(milliseconds to wait=u32 10) -> ()  [unwired: 1 out]
        n1413 = call-poly "VISA Configure Serial Port"("VISA resource name"=refnum<visa-resource-name> "ASRL1::INSTR" ("COM PORT"), "timeout (10sec)"=u32 10, "baud rate (9600)"=u32 57600, "data bits (8)"=u16 8, "stop bits (10: 1 bit)"=w1569) -> ("VISA resource name out"=w1555:refnum<visa-resource-name>, "error out"=w1564:errorcluster)  [unwired: 9 in]
        n1414 = VISA Read(VISA resource name=w1555, byte count=u32 2 ("byte count (0)")) -> (read buffer=w1563:string)  [unwired: 1 in, 3 out]
        n1415 = String Subset(string=w1563, offset (0)=0, length (rest)=2 ("length (rest)")) -> (substring=w1562:string)
        n1416 = Match Pattern(string=w1562, regular expression="<>") -> (offset past match=w1559:i32)  [unwired: 1 in, 3 out]
        n1417 = Greater Or Equal?(x=w1559, y=0) -> (x >= y?=w1554:bool)
        n1418 = case shown="True" w1554 {
          tunnel: w1555 -> [_ w1573]
          tunnel: w1564 -> [_ w1572]
          frame False {
          }
          frame True {
            n1419 = VISA Read(VISA resource name=w1573, byte count=u32 32 ("byte count (0)"), error in (no error)=w1572) -> (read buffer=w1571:string)  [unwired: 3 out]
            n1420 = String Subset(string=w1571, offset (0)=0, length (rest)=8 ("length (rest)")) -> (substring=w1575:string)
            n1421 = String Subset(string=w1571, offset (0)=8, length (rest)=8 ("length (rest)")) -> (substring=w1576:string)
            n1422 = Decimal String To Number(string=w1576) -> (number=w1583:i32)  [unwired: 2 in, 1 out]
            n1423 = Decimal String To Number(string=w1575) -> (number=w1579:i32)  [unwired: 2 in, 1 out]
            n1424 = Divide(x=w1583, y=10000) -> ()  [unwired: 1 out]
            n1425 = Divide(x=w1579, y=1000000) -> ()  [unwired: 1 out]
          }
        }
        n1426 = local read "Quit"() -> (w1552:bool)
      }
    }
    frame Enabled {
    }
  }
  n1427 = while {
    stop <- w1587 stop-if-true
    n1428 = local read "Error  2"() -> (w1585:errorcluster)
    n1429 = case shown="No Error" w1585 {
      frame No Error {
        n1430 = local read "Read Humidity"() -> (w1588:string)
        n1431 = String To Byte Array(string=w1588) -> (unsigned byte array=w1594:u8[])
        n1432 = Array Size(array=w1594) -> (size(s)=w1593:i32)
        n1433 = formula code="// 1. Declare ALL internal variables at the very top (using 'int' and 'float')\nint i = 0;\nint k = 0;\nint start_idx = -1;\nint end_idx = -1;\nint phase = 0;\nint sign0 = 1;\nint sign1 = 1;\nint ch0_val = 0;   \nint ch1_val = 0;   \nfloat ch0_raw = 0.0;\nfloat ch1_raw = 0.0;\n\n// Initialize tracking variables using 'float'\nfloat max_ch0 = -9999999.0;\nfloat min_ch0 =  9999999.0;\nfloat max_ch1 = -9999999.0;\nfloat min_ch1 =  9999999.0;\n\n// Default outputs to 0\nvalid_data = 0;\nLVDT_Min_V = 0.0; LVDT_Max_V = 0.0; LVDT_P2P_V = 0.0;\nPiezo_P2P = 0.0; Friction_N = 0.0; COF = 0.0;\n\n// Scan the byte array for packets\nfor (i = 0; i < array_size - 1; i++) {\n    // Look for the start delimiter '*' (ASCII 42)\n    if (raw_bytes[i] == 42) {\n        start_idx = i;\n    }\n    \n    // Look for the end delimiter ';&' (ASCII 59 and 38)\n    if (raw_bytes[i] == 59 && raw_bytes[i+1] == 38 && start_idx != -1) {\n        end_idx = i;\n        ch0_val = 0;\n        ch1_val = 0;\n        sign0 = 1;\n        sign1 = 1;\n        phase = 0; // 0 = parsing Ch0, 1 = parsing Ch1\n\n        // Parse ASCII characters inside this specific packet frame\n        for (k = start_idx + 1; k < end_idx; k++) {\n            if (raw_bytes[k] == 45) { // Negative sign '-'\n                if (phase == 0) sign0 = -1;\n                else sign1 = -1;\n            }\n            else if (raw_bytes[k] == 59) { // Separator ';'\n                phase = 1; \n            }\n            else if (raw_bytes[k] >= 48 && raw_bytes[k] <= 57) { // Numbers '0'-'9'\n                if (phase == 0) {\n                    ch0_val = (ch0_val * 10) + (raw_bytes[k] - 48);\n                } else {\n                    ch1_val = (ch1_val * 10) + (raw_bytes[k] - 48);\n                }\n            }\n        }\n\n        // FIXED: Removed the C-style (float) cast syntax. LabVIEW auto-promotes this seamlessly.\n        ch0_raw = ch0_val * sign0;\n        ch1_raw = ch1_val * sign1;\n        valid_data = 1;\n\n        // Track Min/Max values across the entire chunk of frames\n        if (ch0_raw > max_ch0) max_ch0 = ch0_raw;\n        if (ch0_raw < min_ch0) min_ch0 = ch0_raw;\n        if (ch1_raw > max_ch1) max_ch1 = ch1_raw;\n        if (ch1_raw < min_ch1) min_ch1 = ch1_raw;\n\n        // Reset start_idx to find the next packet in the loop\n        start_idx = -1; \n    }\n}\n\n// Step 2: If valid packets were parsed, calculate physical metrics using user entries\nif (valid_data == 1) {\n    // LVDT Scaling\n    LVDT_Min_V = (min_ch0 * VREF) / ADC_Resolution;\n    LVDT_Max_V = (max_ch0 * VREF) / ADC_Resolution;\n    LVDT_P2P_V = LVDT_Max_V - LVDT_Min_V;\n\n    // Piezo, Friction & COF Scaling\n    Piezo_P2P = max_ch1 - min_ch1;\n    Friction_N = Piezo_P2P * PIEZO_CAL_FACTOR;\n    COF = Friction_N / NORMAL_FORCE;\n}"("raw_bytes"=w1594, "array_size"=w1593, "VREF"="VREF", "ADC_Resolution"="ADC_Resolution", "PIEZO_CAL_FACTOR"="PIEZO_CAL_FACTOR", "NORMAL_FORCE"="NORMAL_FORCE") -> ("valid_data"=→"Valid_data":dbl, "LVDT_Min_V"=→"LVDT MIN":dbl, "LVDT_Max_V"=→"LVDT MAX":dbl, "LVDT_P2P_V"=→"LVDT Peak":dbl, "Piezo_P2P"=→"pizo raw":dbl, "Friction_N"=→"Friction":dbl, "COF"=→"cof":dbl)
      }
      frame Error {
      }
    }
    n1434 = Wait (ms)(milliseconds to wait=u32 40) -> ()  [unwired: 1 out]
    n1435 = local read "Quit"() -> (w1587:bool)
  }
  n1436 = disable-structure shown="Disabled" {
    disable-tunnel: errorcluster {"status"=TRUE, "code"=0, "source"="Init"} ("error IO") -> [w1604 _]
    disable-tunnel: [w1602 _] -> w44
    frame Disabled {
      n1437 = while {
        shift-right: [w1620] -> w1606
        shift-left: _ -> [w1611]
        shift-right: [w1619] -> w1605
        shift-left: w1604 -> [w1613]
        tunnel: [w1608] -> w1602
        tunnel: [w1618] -> _
        i -> [w1618]
        stop <- w1608 stop-if-true
        n1438 = local read "Port 1a"() -> (w1614:bool)
        n1439 = local read "Port 3"() -> (w1615:bool)
        n1440 = local read "Com Port 1"() -> (w1612:refnum<visa-resource-name>)
        n1441 = Or(x=w1615, y=w1614) -> (x .or. y?=w1617:bool)
        n1442 = Unbundle(w1613) -> ("status"=→"Port 3":bool)  [unwired: 2 out]
        n1443 = Not Equal?(x=w1612, y=w1611) -> (x != y?=w1609:bool)
        n1444 = case shown="True" w1617 {
          frame False {
            w1623 = TRUE ("Visible")
            n1445 = property on="Port 1a" class="Bool (strict)"("Visible"=w1623) -> ()  [unwired: 2 in, 2 out]
            n1446 = property on="Port 3" class="Bool (strict)"("Visible"=w1623) -> ()  [unwired: 2 in, 2 out]
          }
          frame True {
            w1624 = TRUE ("Visible")
            n1447 = property on="Port 1a" class="Bool (strict)"("Visible"=w1624) -> ()  [unwired: 2 in, 2 out]
            n1448 = property on="Port 3" class="Bool (strict)"("Visible"=w1624) -> ()  [unwired: 2 in, 2 out]
          }
        }
        n1449 = Wait (ms)(milliseconds to wait=u32 40) -> ()  [unwired: 1 out]
        n1450 = case shown="True" w1609 {
          tunnel: [w1621 errorcluster {"status"=TRUE, "code"=0, "source"="Init"} ("error out")] -> w1610
          tunnel: w1613 -> [w1621 _]
          frame False {
          }
          frame True {
          }
        }
        "error out 11" <- w1610
        n1451 = case shown="No Error" w1610 {
          selector: w1610 -> [w1631 w1649]
          tunnel: [w1634 w1653] -> w1620
